vi "build_graph-vertical.vi"(8 "error in (no error)":errorcluster, 10 "y_axis":dbl[][](array[numeric]), 11 "x_axis":dbl[](array[numeric])) -> (0 "error out":errorcluster, 4 "graph_data":T2(array[cluster]), 6 "scale_ranges":T1)   [LabVIEW 2015, in "lv-graph.lvlib"]
uses:
  lv-graph.lvlib
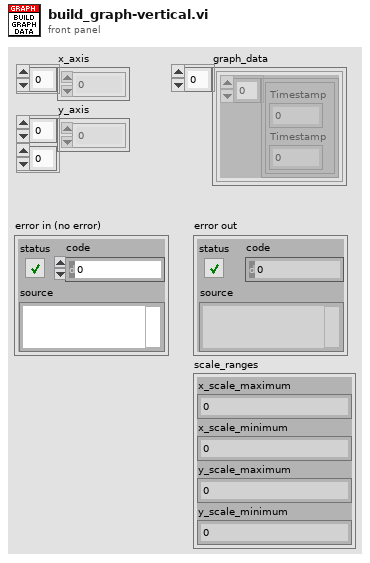
[diagram p1: front panel]
types:
  T1 = cluster{"x_scale_maximum":dbl, "x_scale_minimum":dbl, "y_scale_maximum":dbl, "y_scale_minimum":dbl}
  T2 = cluster{cluster{"Timestamp":dbl, "Timestamp":dbl}[]}[]
  T3 = cluster{cluster{"Timestamp":dbl, "Timestamp":dbl}[]}
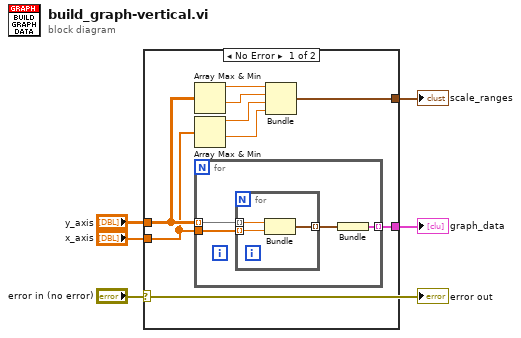
[diagram p0: block diagram]
diagram:
  n1 = case shown="No Error" "error in (no error)" {
    tunnel: [w13 _] -> w3
    tunnel: "y_axis" -> [w7 _]
    tunnel: "x_axis" -> [w6 _]
    tunnel: [w8 _] -> w2
    frame No Error {
      n2 = Array Max & Min(array=w7) -> (max value=w10:dbl, min value=w9:dbl)  [unwired: 2 out]
      n3 = Array Max & Min(array=w6) -> (max value=w11:dbl, min value=w12:dbl)  [unwired: 2 out]
      n4 = for {
        tunnel: [w15] -> w13 mode=indexing
        tunnel: w7 -> [w17] mode=indexing
        tunnel: w6 -> [w16]
        n5 = for {
          tunnel: w16 -> [w18] mode=indexing
          tunnel: w17 -> [w19] mode=indexing
          tunnel: [w20] -> w14 mode=indexing
          n6 = Bundle("Timestamp"=w19, "Timestamp"=w18) -> (w20:cluster{"Timestamp":dbl, "Timestamp":dbl})  [unwired: 1 in]
        }
        n7 = Bundle(w14) -> (w15:T3)  [unwired: 1 in]
      }
      n8 = Bundle(w10, w9, w11, w12) -> (w8:cluster{dbl, dbl, dbl, dbl})  [unwired: 1 in]
    }
    frame Error {
    }
  }
  "graph_data" <- w3
  "scale_ranges" <- w2
  "error out" <- "error in (no error)"
